vi "Move Contained Files to Folder.vi"(6 "exclued files":string[](array[string]), 8 "error in (no error)":errorcluster, 10 "Dest Foder Path":path, 11 "Folder Path":path) -> (0 "error out":errorcluster)   [LabVIEW 2017, in "FileSync -- Base.lvlib" / "Protocol.lvclass"]
uses:
  Protocol.lvclass
  <userlib>/_OpenG.lib/file/file.llb/Compare Two Paths - Scalar__ogtk.vi
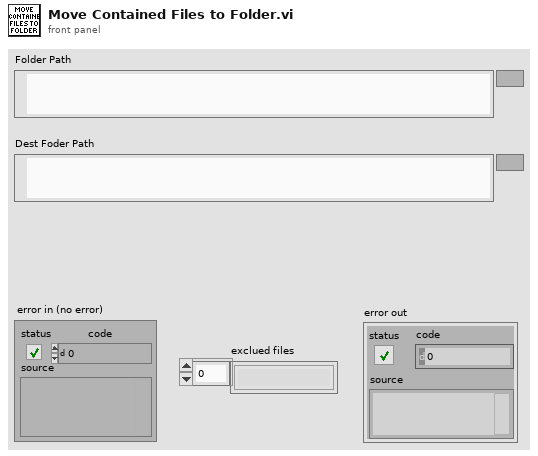
[diagram p1: front panel]
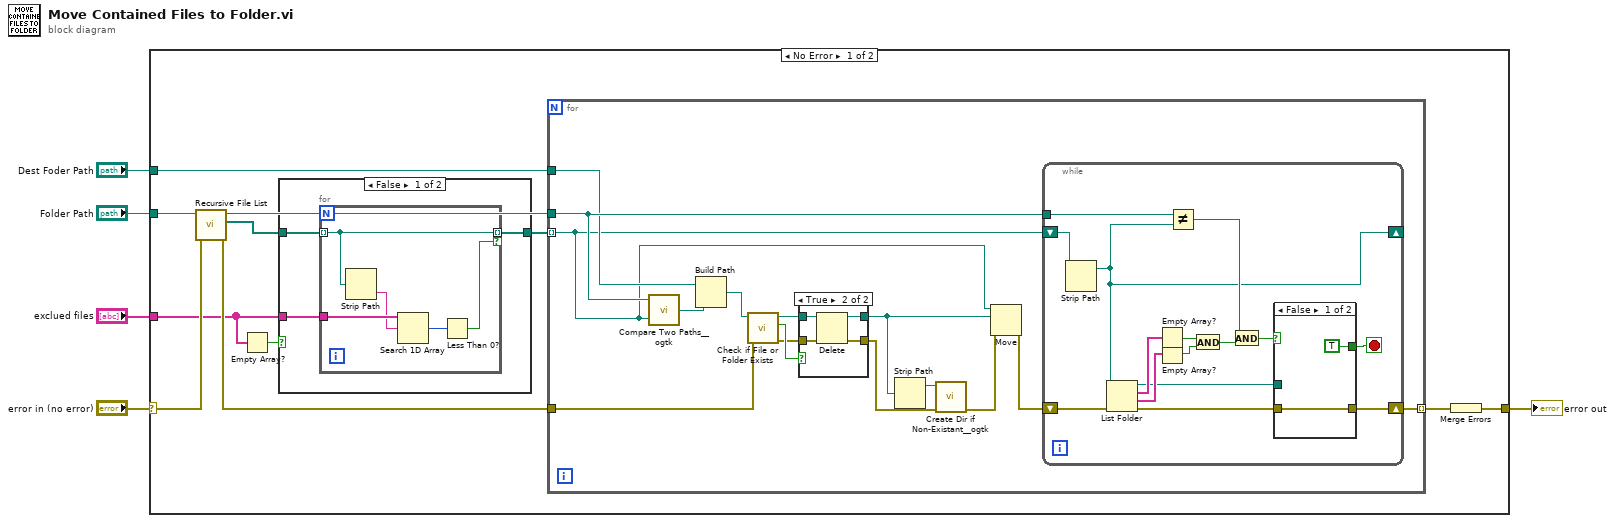
[diagram p0: block diagram]
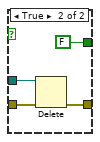
[diagram p3: hidden frame]
diagram:
  n1 = case shown="No Error" "error in (no error)" {
    selector: "error in (no error)" -> [w16 w68]
    tunnel: "Folder Path" -> [w14 _]
    tunnel: "Dest Foder Path" -> [w13 _]
    tunnel: [w10 w68] -> w2
    tunnel: "exclued files" -> [w9 _]
    frame No Error {
      n2 = call <vilib>:"Recursive File List.vi"("error in (no error)"=w16, "Folder Path"=w14) -> ("error out"=w15:errorcluster, "All Files in Dir"=w7:path[], "dup Folder Path"=w12:path)  [unwired: 5 in, 2 out]
      n3 = Empty Array?(array=w9) -> (empty?=w8:bool)
      n4 = case shown="False" w8 {
        tunnel: w9 -> [w19 _]
        tunnel: w7 -> [w18 w25]
        tunnel: [w17 w25] -> w6
        frame False {
          n5 = for {
            tunnel: w19 -> [w24]
            tunnel: w18 -> [w23] mode=indexing
            tunnel: [w23] -> w17 mode=indexing if=w20
            n6 = Strip Path(path=w23) -> (name=w22:string)  [unwired: 1 out]
            n7 = Search 1D Array(1D array=w24, element=w22) -> (index of element=w21:i32)  [unwired: 1 in]
            n8 = Less Than 0?(x=w21) -> (x < 0?=w20:bool)
          }
        }
        frame True {
        }
      }
      n9 = for {
        tunnel: w6 -> [w26] mode=indexing
        tunnel: w15 -> [w40]
        tunnel: w13 -> [w29]
        tunnel: w12 -> [w30]
        tunnel: [w27] -> w11 mode=indexing
        n10 = call-poly <userlib>:"Compare Two Paths__ogtk.vi"("path2"=w26, "path1"=w30) -> ("relative path from 1 to 2"=w39:path)  [unwired: 1 in, 2 out]
        n11 = Build Path(base path=w29, name or relative path=w39) -> (appended path=w38:path)
        n12 = call <vilib>:"Check if File or Folder Exists.vi"("error in (no error)"=w40, "path"=w38) -> ("error out"=w35:errorcluster, "file or folder exists?"=w36:bool, "dup path"=w37:path)  [unwired: 7 in]
        n13 = case shown="True" w36 {
          tunnel: w37 -> [w63 w67]
          tunnel: [w63 w66] -> w34
          tunnel: w35 -> [w62 w65]
          tunnel: [w62 w64] -> w32
          frame False {
          }
          frame True {
            n14 = Delete(path (use dialog)=w67, error in=w65) -> (deleted path=w66:path, error out=w64:errorcluster)  [unwired: 3 in, 1 out]
          }
        }
        n15 = Strip Path(path=w34) -> (stripped path=w33:path)  [unwired: 1 out]
        n16 = call <userlib>:"Create Dir if Non-Existant__ogtk.vi"("error in (no error)"=w32, "Directory Path"=w33) -> ("error out"=w31:errorcluster)  [unwired: 7 in, 2 out]
        n17 = Move(source path=w26, error in=w31, 10:w34) -> (error out=w28:errorcluster)  [unwired: 2 in, 2 out]
        n18 = while {
          tunnel: w30 -> [w47]
          shift-right: [w43] -> w27
          shift-left: w28 -> [w44]
          shift-right: [w42] -> _
          shift-left: w26 -> [w48]
          stop <- w41 stop-if-true
          n19 = Strip Path(path=w48) -> (stripped path=w42:path)  [unwired: 1 out]
          n20 = List Folder(path=w42, error in=w44) -> (path out=w49:path, filenames=w55:string[], folder names=w54:string[], error out=w46:errorcluster)  [unwired: 2 in]
          n21 = Empty Array?(array=w55) -> (empty?=w53:bool)
          n22 = Empty Array?(array=w54) -> (empty?=w52:bool)
          n23 = Not Equal?(x=w47, y=w42) -> (x != y?=w50:bool)
          n24 = And(x=w53, y=w52) -> (x .and. y?=w51:bool)
          n25 = And(x=w50, y=w51) -> (x .and. y?=w45:bool)
          n26 = case shown="False" w45 {
            tunnel: w49 -> [_ w61]
            tunnel: w46 -> [w57 w60]
            tunnel: [w57 w59] -> w43
            tunnel: [TRUE FALSE] -> w41
            frame False {
            }
            frame True {
              n27 = Delete(path (use dialog)=w61, error in=w60) -> (error out=w59:errorcluster)  [unwired: 3 in, 2 out]
            }
          }
        }
      }
      n28 = Merge Errors(w11) -> (w10:errorcluster)
    }
    frame Error {
    }
  }
  "error out" <- w2
